vi "myRIO_BRig_Host_v0,10.vi"() -> ()   [LabVIEW 2014]
panel:
  out "RunTime_minutes":u16
  out "RunTime_seconds":u16
  out "error out 2":errorcluster caption="error out"
  in  "dataIn_maxTrialsDisplayed":u16 caption="Number of Trials Displayed\n( 0 = all trials )"
  in  "colorIn_timeout":u32(colorbox)=7468543 caption="Choice Timeout"
  in  "colorIn_wrong/cue":u32(colorbox)=16728618 caption="Wrong Choice or\nLicked During Cue"
  in  "colorIn_reward":u32(colorbox)=5898088 caption="Reward"
  in  "colorIn_unknown":u32(colorbox)=16449331 caption="Unknown Trial Status"
  in  "LoadPrevSettings":bool
  out "BlockL_BTPR_cur":u16 caption="BadTrialsPostReward"
  out "BlockL_T2R_cur":u16 caption="Trials2Reward"
  out "BlockL_BTPR_avg":dbl caption="BadTrialsPostReward" format="%#_3g"
  out "BlockL_T2R_avg":dbl caption="Trials2Reward" format="%#_3g"
  out "BlockR_BTPR_cur":u16 caption="BadTrialsPostReward"
  out "BlockR_T2R_cur":u16 caption="Trials2Reward"
  out "BlockR_BTPR_avg":dbl caption="BadTrialsPostReward" format="%#_3g"
  out "BlockR_T2R_avg":dbl caption="Trials2Reward" format="%#_3g"
  out "dataOut_plot":cluster{i32[], i32[]}[](graph)
  out "iBlock":u16
  out "iTrial":u16
  in  "stop":bool
  # "Exp Stats"
  # "Current Block Stats"
  # "Trials 2 Reward\n\nBad Trials\nPost Reward"
  # "Left Spout    Right Spout"
  # "Run Time\n\n   minutes    seconds"
  # "Average Block Stats"
  # "Trials 2 Reward\n\nBad Trials\nPost Reward"
  # "Left Spout    Right Spout"
  # "If you get ERROR 5 related to opening a file, press CONTINUE"
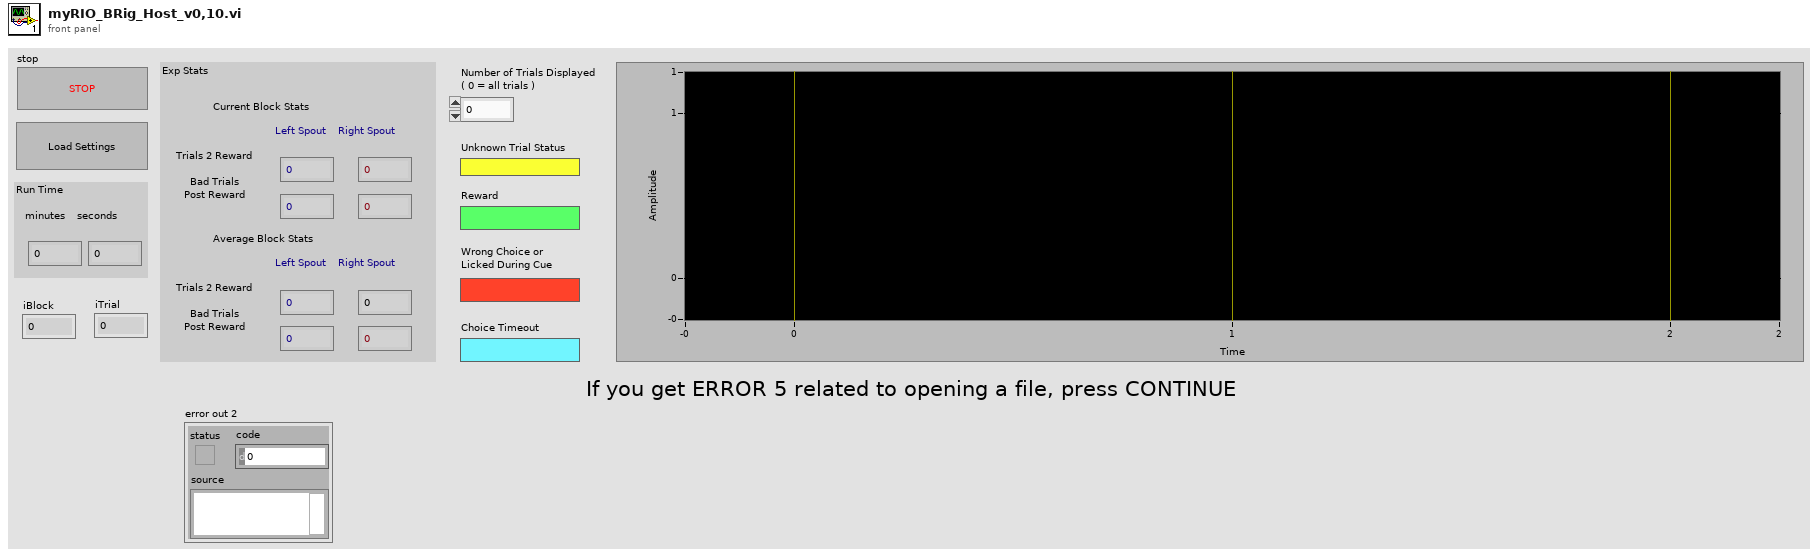
[diagram p1: front panel]
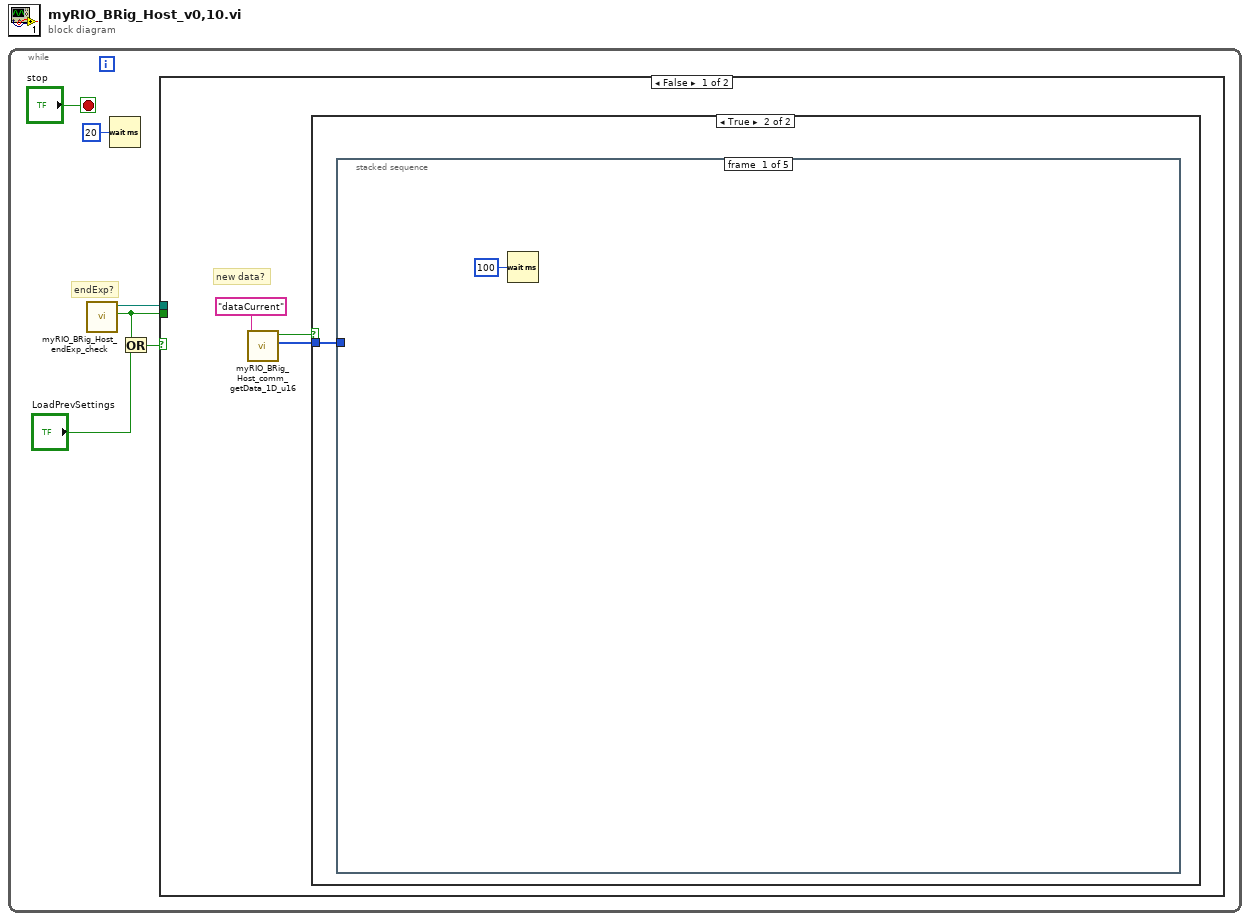
[diagram p0: block diagram]
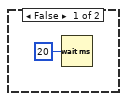
[diagram p2: hidden frame]
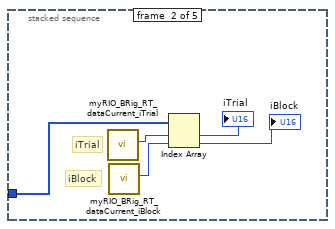
[diagram p3: hidden frame]
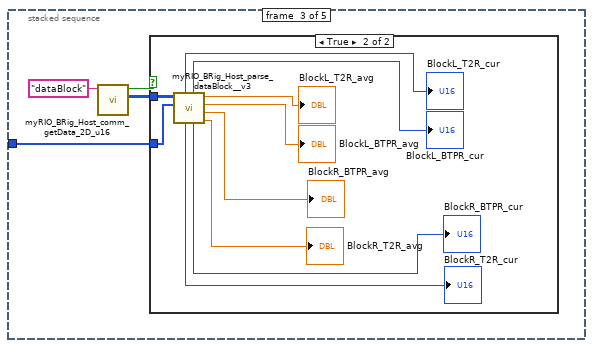
[diagram p4: hidden frame]
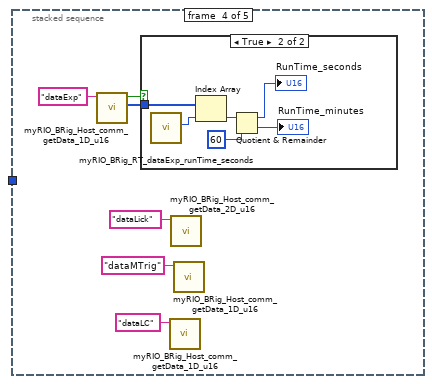
[diagram p6: hidden frame]
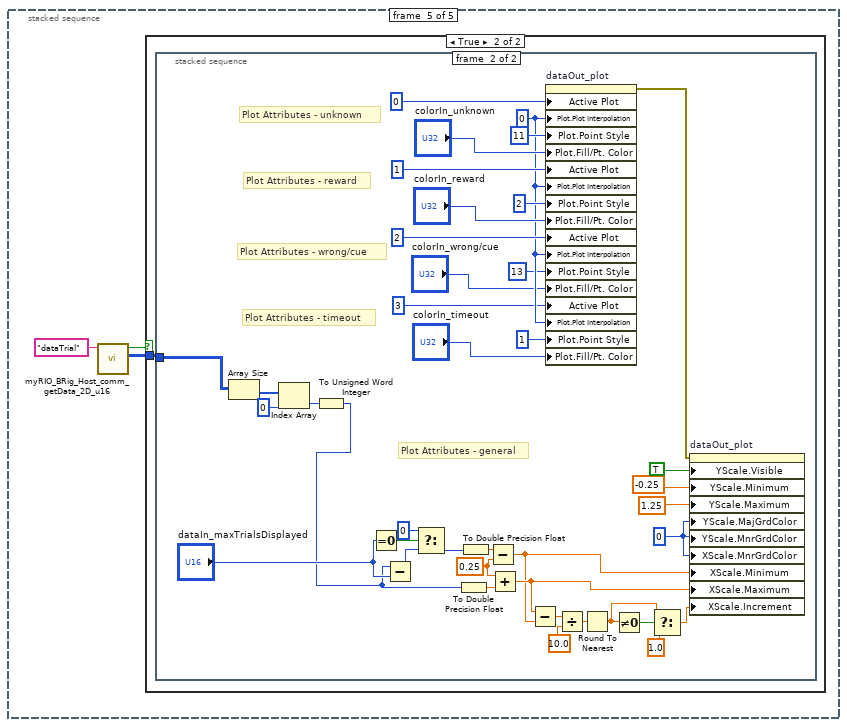
[diagram p8: hidden frame]
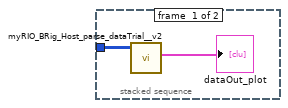
[diagram p10: hidden frame]
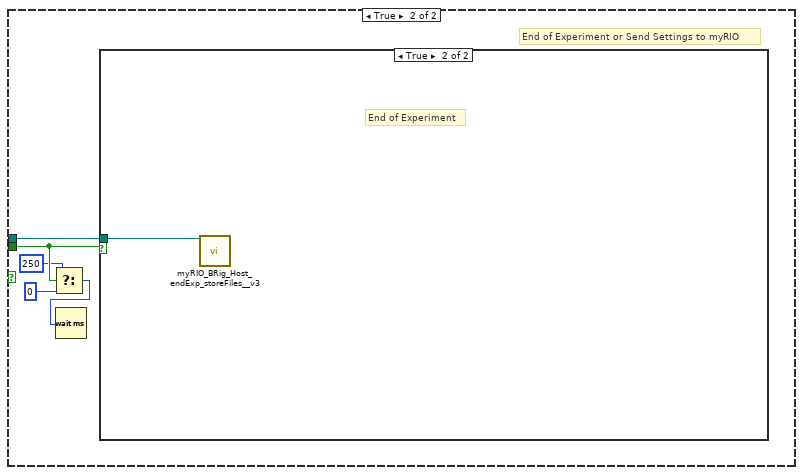
[diagram p11: hidden frame]
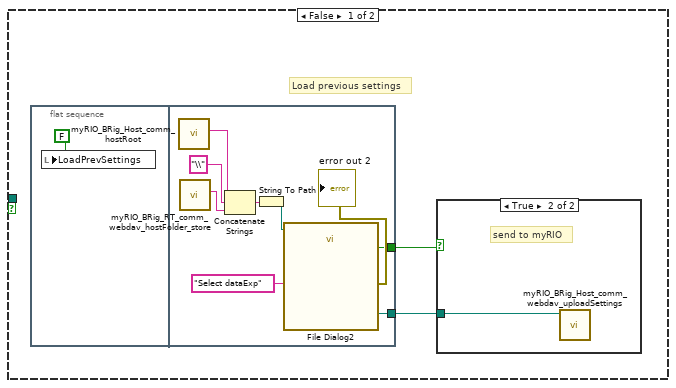
[diagram p12: hidden frame]
diagram:
  n1 = while {
    stop <- "stop" stop-if-true
    # "endExp?"
    n2 = call "myRIO_BRig_Host_endExp_check.vi"() -> ("output_IendExp"=w3:bool, "output_filePath_expExp"=w2:path)  [unwired: 10 in]
    n3 = Wait (ms)(milliseconds to wait=u32 20) -> ()  [unwired: 1 out]
    n4 = Or(x=w3, y="LoadPrevSettings") -> (x .or. y?=w4:bool)
    n5 = case shown="False" w4 {
      tunnel: w3 -> [_ w93]
      tunnel: w2 -> [_ w94]
      frame False {
        # "new data?"
        n6 = call "myRIO_BRig_Host_comm_getData_1D_u16.vi"("input_fileName"="dataCurrent") -> ("output_data_1D"=w7:u16[], "output_I_data"=w8:bool)  [unwired: 9 in]
        n7 = case shown="True" w8 {
          tunnel: w7 -> [_ w11]
          frame False {
            n8 = Wait (ms)(milliseconds to wait=u32 20) -> ()  [unwired: 1 out]
          }
          frame True {
            n9 = stacked-sequence {
              tunnel: w11 -> [_ w13 w18 _ _]
              frame #0 {
                n10 = Wait (ms)(milliseconds to wait=u32 100) -> ()  [unwired: 1 out]
              }
              frame #1 {
                # "iBlock"
                # "iTrial"
                n11 = call "myRIO_BRig_RT_dataCurrent_iTrial.vi"() -> ("output_iTrial"=w17:i32)  [unwired: 11 in]
                n12 = call "myRIO_BRig_RT_dataCurrent_iBlock.vi"() -> ("output_iBlock"=w16:i32)  [unwired: 11 in]
                n13 = Index Array(array=w13, index #1=w17, index #2=w16) -> (element #1=→"iTrial":u16, element #2=→"iBlock":u16)
              }
              frame #2 {
                n14 = call "myRIO_BRig_Host_comm_getData_2D_u16.vi"("input_fileName"="dataBlock") -> ("output_data_2D"=w19:u16[][], "output_I_data"=w20:bool)  [unwired: 9 in]
                n15 = case shown="True" w20 {
                  tunnel: w19 -> [_ w23]
                  tunnel: w18 -> [_ w22]
                  frame False {
                  }
                  frame True {
                    n16 = call "myRIO_BRig_Host_parse_dataBlock__v3.vi"("input_dataCurrent"=w22, "input_dataBlock"=w23) -> ("BlockR_T2R_avg"=→"BlockR_T2R_avg":dbl, "BlockR_BTPR_avg"=→"BlockR_BTPR_avg":dbl, "BlockL_BTPR_avg"=→"BlockL_BTPR_avg":dbl, "BlockL_T2R_avg"=→"BlockL_T2R_avg":dbl, "BlockR_BTPR_cur"=→"BlockR_BTPR_cur":u16, "BlockL_BTPR_cur"=→"BlockL_BTPR_cur":u16, "BlockR_T2R_cur"=→"BlockR_T2R_cur":u16, "BlockL_T2R_cur"=→"BlockL_T2R_cur":u16)  [unwired: 2 in]
                  }
                }
              }
              frame #3 {
                n17 = call "myRIO_BRig_Host_comm_getData_1D_u16.vi"("input_fileName"="dataExp") -> ("output_data_1D"=w35:u16[], "output_I_data"=w36:bool)  [unwired: 9 in]
                n18 = case shown="True" w36 {
                  tunnel: w35 -> [_ w43]
                  frame False {
                  }
                  frame True {
                    n19 = call "myRIO_BRig_RT_dataExp_runTime_seconds.vi"() -> ("output_RunTime_minutes"=w42:i32)  [unwired: 11 in]
                    n20 = Index Array(array=w43, index=w42) -> (element=w41:u16)
                    n21 = Quotient & Remainder(x=w41, y=u16 60) -> (x-y*floor(x/y)=→"RunTime_seconds":u16, floor(x/y)=→"RunTime_minutes":u16)
                  }
                }
                n22 = call "myRIO_BRig_Host_comm_getData_1D_u16.vi"("input_fileName"="dataLC") -> ()  [unwired: 9 in, 2 out]
                n23 = call "myRIO_BRig_Host_comm_getData_2D_u16.vi"("input_fileName"="dataLick") -> ()  [unwired: 9 in, 2 out]
                n24 = call "myRIO_BRig_Host_comm_getData_1D_u16.vi"("input_fileName"="dataMTrig") -> ()  [unwired: 9 in, 2 out]
              }
              frame #4 {
                n25 = call "myRIO_BRig_Host_comm_getData_2D_u16.vi"("input_fileName"="dataTrial") -> ("output_data_2D"=w45:u16[][], "output_I_data"=w44:bool)  [unwired: 9 in]
                n26 = case shown="True" w44 {
                  tunnel: w45 -> [_ w47]
                  frame False {
                  }
                  frame True {
                    n27 = stacked-sequence {
                      tunnel: w47 -> [w48 w54]
                      frame #0 {
                        n28 = call "myRIO_BRig_Host_parse_dataTrial__v2.vi"("arrayIn_dataTrial"=w48) -> ("appended array"=→"dataOut_plot":cluster{i32[], i32[]}[])  [unwired: 10 in]
                      }
                      frame #1 {
                        w69 = 0.25 ("y")
                        w73 = u32 0 ("Y Scale.Grid Colors:Major Color")
                        w82 = u8 0 ("Plot.Plot Interpolation")
                        # "Plot Attributes - general"
                        # "Plot Attributes - timeout"
                        # "Plot Attributes - wrong/cue"
                        # "Plot Attributes - reward"
                        # "Plot Attributes - unknown"
                        n29 = Array Size(array=w54) -> (size(s)=w56:i32[])
                        n30 = Index Array(array=w56, index=0) -> (element=w52:i32)
                        n31 = To Unsigned Word Integer(number=w52) -> (unsigned 16bit integer=w51:u16)
                        n32 = Equal To 0?(x="dataIn_maxTrialsDisplayed") -> (x = 0?=w72:bool)
                        n33 = Subtract(x=w51, y="dataIn_maxTrialsDisplayed") -> (x-y=w71:u16)
                        n34 = Select(t=u16 0, s=w72, f=w71) -> (s? t:f=w66:u16)
                        n35 = To Double Precision Float(number=w51) -> (double precision float=w68:dbl)
                        n36 = To Double Precision Float(number=w66) -> (double precision float=w67:dbl)
                        n37 = Subtract(x=w67, y=w69) -> (x-y=w58:dbl)
                        n38 = Add(x=w69, y=w68) -> (x+y=w59:dbl)
                        n39 = Subtract(x=w59, y=w58) -> (x-y=w65:dbl)
                        n40 = property on="dataOut_plot" class="XYGraph (strict)"("Active Plot"=u32 0, "Plot.Plot Interpolation"=w82, "Plot.Point Style"=u8 11, "Plot.Fill/Pt. Color"="colorIn_unknown", "Active Plot"=u32 1, "Plot.Plot Interpolation"=w82, "Plot.Point Style"=u8 2, "Plot.Fill/Pt. Color"="colorIn_reward", "Active Plot"=u32 2, "Plot.Plot Interpolation"=w82, "Plot.Point Style"=u8 13, "Plot.Fill/Pt. Color"="colorIn_wrong/cue", "Active Plot"=u32 3, "Plot.Plot Interpolation"=w82, "Plot.Point Style"=u8 1, "Plot.Fill/Pt. Color"="colorIn_timeout") -> (error out=w57:errorcluster)  [unwired: 2 in, 1 out]
                        n41 = Divide(x=w65, y=10.0) -> (x/y=w63:dbl)
                        n42 = Round To Nearest(number=w63) -> (nearest integer value=w61:dbl)
                        n43 = Not Equal To 0?(x=w61) -> (x != 0?=w62:bool)
                        n44 = Select(t=w61, s=w62, f=1.0) -> (s? t:f=w60:dbl)
                        n45 = property on="dataOut_plot" class="XYGraph (strict)"(error in=w57, "YScale.Visible"=TRUE ("Y Scale.Visible"), "YScale.Minimum"=-0.25 ("Y Scale.Range:Minimum"), "YScale.Maximum"=1.25 ("Y Scale.Range:Maximum"), "YScale.MajGrdColor"=w73, "YScale.MnrGrdColor"=w73, "XScale.MnrGrdColor"=w73, "XScale.Minimum"=w58, "XScale.Maximum"=w59, "XScale.Increment"=w60) -> ()  [unwired: 1 in, 2 out]
                      }
                    }
                  }
                }
              }
            }
          }
        }
      }
      frame True {
        # "End of Experiment or Send Settings to myRIO"
        n46 = Select(t=u32 250 ("milliseconds to wait"), s=w93, f=u32 0 ("milliseconds to wait")) -> (s? t:f=w91:u32)
        n47 = Wait (ms)(milliseconds to wait=w91) -> ()  [unwired: 1 out]
        n48 = case shown="True" w93 {
          tunnel: w94 -> [_ w108]
          frame False {
            # "Load previous settings"
            n49 = flat-sequence {
              tunnel: [w100] -> w95
              tunnel: [w99] -> w96
              frame #0 {
                n50 = local write "LoadPrevSettings"(FALSE ("LoadPrevSettings")) -> ()
              }
              frame #1 {
                n51 = call "myRIO_BRig_Host_comm_hostRoot.vi"() -> ("output_hostRoot"=w102:string)  [unwired: 11 in]
                n52 = call "myRIO_BRig_RT_comm_webdav_hostFolder_store.vi"() -> ("output_HostFolder"=w104:string)  [unwired: 11 in]
                n53 = Concatenate Strings(w102, "\\" ("string"), w104) -> (w106:string)
                n54 = String To Path(string=w106) -> (path=w105:path)
                n55 = call "File Dialog2"("start path"=w105, "prompt"="Select dataExp") -> ("selected path"=w100:path, "exists"=w99:bool, "error out"=→"error out 2":errorcluster)  [unwired: 10 in, 1 out]
              }
            }
            n56 = case shown="True" w96 {
              tunnel: w95 -> [_ w97]
              frame False {
                # "invalid file\nor\ncancelled"
              }
              frame True {
                # "send to myRIO"
                n57 = call "myRIO_BRig_Host_comm_webdav_uploadSettings.vi"("input_filePath"=w97) -> ()  [unwired: 11 in]
              }
            }
          }
          frame True {
            # "End of Experiment"
            n58 = call "myRIO_BRig_Host_endExp_storeFiles__v3.vi"("input_filePath"=w108) -> ()  [unwired: 15 in]
          }
        }
      }
    }
  }
